vi "Open thermocouple VI 2.vi"(8 "Signaller in":refnum<class "Signaller.lvclass">, 10 "chart_temp ref":refnum<vi>, 11 "Temperaturs":refnum<vi>) -> ()   [LabVIEW 2019]
uses:
  Simulation/Signaller/Signaller.lvclass
panel:
  out "format string":string
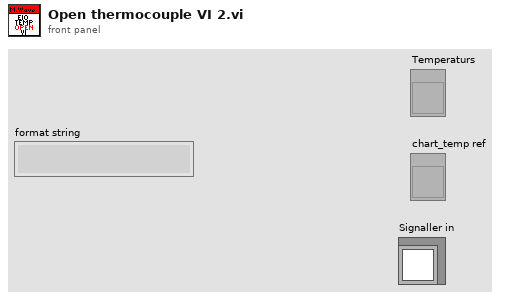
[diagram p1: front panel]
types:
  T1 = enum32{"Bad", "Idle", "Run top level", "Running"}
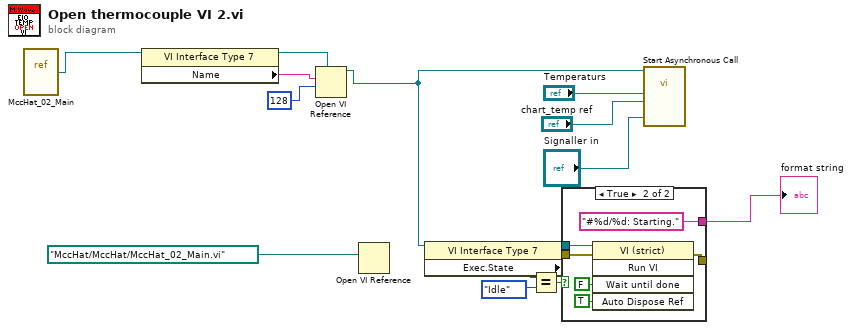
[diagram p0: block diagram]
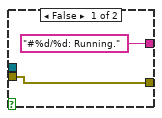
[diagram p2: hidden frame]
diagram:
  n1 = vi-ref "MccHat_02_Main.vi"() -> (w6:refnum<vi>)
  n2 = property class="VI Interface Type 7"(reference=w6) -> (reference out=w5:refnum<vi>, "Name"=w8:string)  [unwired: 1 in, 1 out]
  n3 = Open VI Reference(type specifier VI Refnum (for type only)=w5, vi path=w8, options=128) -> (vi reference=w4:refnum<vi>)  [unwired: 3 in, 1 out]
  n4 = Open VI Reference(vi path=path "MccHat/MccHat/MccHat_02_Main.vi") -> ()  [unwired: 5 in, 2 out]
  n5 = property class="VI Interface Type 7"(reference=w4) -> (reference out=w15:refnum<vi>, error out=w14:errorcluster, "Exec.State"=w13:T1)  [unwired: 1 in]
  n6 = Equal?(x=w13, y=T1."Idle" ("Execution:State")) -> (x = y?=w11:bool)
  n7 = case shown="True" w11 {
    tunnel: w15 -> [_ w21]
    tunnel: w14 -> [w17 w20]
    tunnel: [w17 w19] -> _
    tunnel: ["#%d/%d: Running." ("format string") "#%d/%d: Starting." ("format string")] -> w9
    frame False {
    }
    frame True {
      n8 = invoke class="VI (strict)" method="Run VI"(reference=w21, error in=w20, "Wait until done"=FALSE ("Wait Until Done"), "Auto Dispose Ref"=TRUE ("Auto Dispose Reference")) -> (error out=w19:errorcluster)  [unwired: 1 in, 4 out]
    }
  }
  "format string" <- w9
  n9 = call-by-ref "Start Asynchronous Call"(reference=w4, "Signaller in"="Signaller in", "chart_temp ref"="chart_temp ref", "Temperaturs"="Temperaturs") -> ()  [unwired: 10 in, 2 out]
